vi "Set Initially Connected Endpoints.vi"(8 "error in (no error)":errorcluster, 10 "Connections":T1[](array[typedef]), 11 "Hardware Ref in":T2 format="%.0x") -> (0 "error out":errorcluster, 3 "Hardware Ref out":T2 format="%.0x")   [LabVIEW 2019, in "Routing and Faulting Hardware API.lvlib"]
doc: "Sets a list of endpoints that are connected when this device is initialized of this instance of a Routing and Faulting Hardware Custom Device"
uses:
  Routing and Faulting Hardware API.lvlib
  <vilib>/NI VeriStand/Custom Device API/Custom Device Item Ref.ctl
  Types/Connection.ctl
  Routing and Faulting Hardware API Constants.vi
  <vilib>/NI VeriStand/Custom Device API/Set Item Property (String Array).vi
  <vilib>/NI VeriStand/Custom Device API/Custom Device API.lvlib
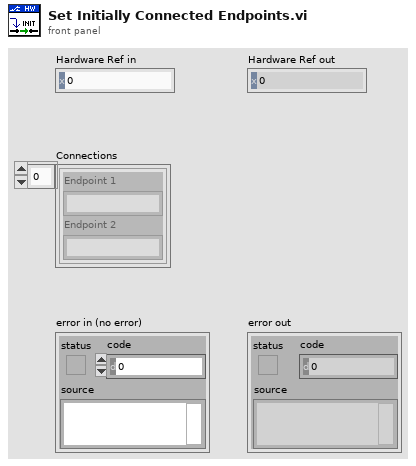
[diagram p1: front panel]
types:
  T1 = typedef "Routing and Faulting Hardware API.lvlib/Connection.ctl" = cluster{"Endpoint 1":string, "Endpoint 2":string}
  T2 = typedef "Custom Device API.lvlib/Custom Device Item Ref.ctl" = u64
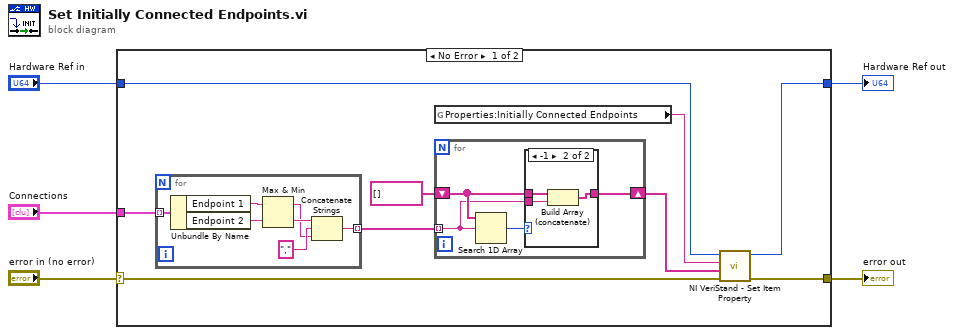
[diagram p0: block diagram]
diagram:
  n1 = case shown="No Error" "error in (no error)" {
    selector: "error in (no error)" -> [w11 w31]
    tunnel: "Hardware Ref in" -> [w14 w30]
    tunnel: [w13 w30] -> w4
    tunnel: [w12 w31] -> w3
    tunnel: "Connections" -> [w9 _]
    frame No Error {
      n2 = for {
        tunnel: w9 -> [w29] mode=indexing
        tunnel: [w23] -> w8 mode=indexing
        n3 = Unbundle By Name(w29) -> ("Endpoint 1"=w28:string, "Endpoint 2"=w27:string)
        n4 = Max & Min(x=w28, y=w27) -> (max(x,y)=w24:string, min(x,y)=w25:string)
        n5 = Concatenate Strings(w25, "," ("string"), w24) -> (w23:string)
      }
      n6 = global read "Routing and Faulting Hardware API Constants.vi" "Properties:Initially Connected Endpoints"() -> (w10:string)
      n7 = for {
        tunnel: w8 -> [w16] mode=indexing
        shift-right: [w17] -> w6
        shift-left: string[] [] -> [w18]
        n8 = Search 1D Array(1D array=w18, element=w16) -> (index of element=w15:i32)  [unwired: 1 in]
        n9 = case shown="-1" w15 {
          tunnel: w18 -> [w19 w22]
          tunnel: [w19 w21] -> w17
          tunnel: w16 -> [_ w20]
          frame Default {
          }
          frame -1 {
            n10 = Build Array (concatenate)(w22, w20) -> (w21:string[])
          }
        }
      }
      n11 = call-poly <vilib>:"NI VeriStand - Set Item Property.vi"("error in (no error)"=w11, "Value"=w6, "Property Name"=w10, "Item Ref in"=w14) -> ("error out"=w12:errorcluster, "Item Ref out"=w13:T2)  [unwired: 5 in, 1 out]
    }
    frame Error {
    }
  }
  "Hardware Ref out" <- w4
  "error out" <- w3
